vi "Word_auto_text_entry (for page number).vi"(0 "Word._Document in":refnum<k7>, 7 "position (footers)":u16(ring) items=["footers", "headers"], 11 "error in (no error)":errorcluster, 12 "alignment (right)":u16(ring)=2 items=["left", "center", "right"]) -> (4 "Word._Document out":refnum<k7>, 15 "error out":errorcluster)   [LabVIEW 2020, in "NI_ReportGenerationToolkit.lvlib"]
uses:
  <vilib>/addons/_office/NI_ReportGenerationToolkit.lvlib
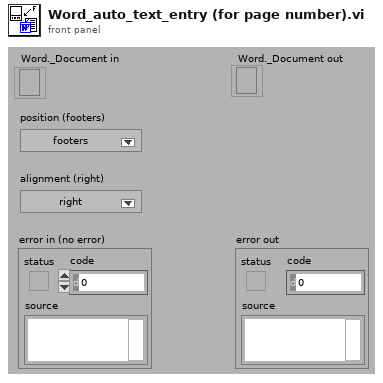
[diagram p1: front panel]
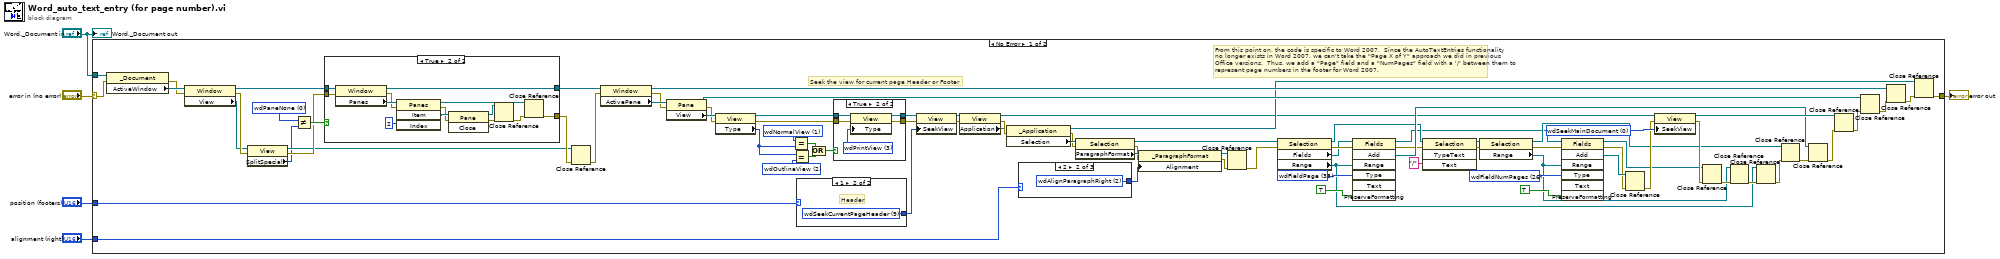
[diagram p0: block diagram]
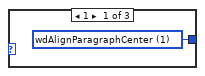
[diagram p2: hidden frame]
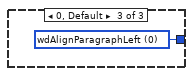
[diagram p3: hidden frame]
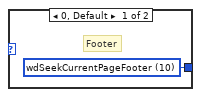
[diagram p4: hidden frame]
diagram:
  n1 = case shown="No Error" "error in (no error)" {
    selector: "error in (no error)" -> [w42 w115]
    tunnel: "Word._Document in" -> [w87 _]
    tunnel: "position (footers)" -> [w58 _]
    tunnel: [w43 w115] -> w4
    tunnel: "alignment (right)" -> [w6 _]
    frame No Error {
      w24 = 26 items=["wdFieldEmpty"=-1, "wdFieldRef"=3, "wdFieldIndexEntry"=4, "wdFieldFootnoteRef"=5, "wdFieldSet"=6, "wdFieldIf"=7, "wdFieldIndex"=8, "wdFieldTOCEntry"=9, "wdFieldStyleRef"=10, "wdFieldRefDoc"=11, "wdFieldSequence"=12, "wdFieldTOC"=13, "wdFieldInfo"=14, "wdFieldTitle"=15, "wdFieldSubject"=16, "wdFieldAuthor"=17, "wdFieldKeyWord"=18, "wdFieldComments"=19, "wdFieldLastSavedBy"=20, "wdFieldCreateDate"=21, "wdFieldSaveDate"=22, "wdFieldPrintDate"=23, "wdFieldRevisionNum"=24, "wdFieldEditTime"=25, "wdFieldNumPages"=26, "wdFieldNumWords"=27, "wdFieldNumChars"=28, "wdFieldFileName"=29, "wdFieldTemplate"=30, "wdFieldDate"=31, "wdFieldTime"=32, "wdFieldPage"=33, "wdFieldExpression"=34, "wdFieldQuote"=35, "wdFieldInclude"=36, "wdFieldPageRef"=37, "wdFieldAsk"=38, "wdFieldFillIn"=39, "wdFieldData"=40, "wdFieldNext"=41, "wdFieldNextIf"=42, "wdFieldSkipIf"=43, "wdFieldMergeRec"=44, "wdFieldDDE"=45, "wdFieldDDEAuto"=46, "wdFieldGlossary"=47, "wdFieldPrint"=48, "wdFieldFormula"=49, "wdFieldGoToButton"=50, "wdFieldMacroButton"=51, "wdFieldAutoNumOutline"=52, "wdFieldAutoNumLegal"=53, "wdFieldAutoNum"=54, "wdFieldImport"=55, "wdFieldLink"=56, "wdFieldSymbol"=57, "wdFieldEmbed"=58, "wdFieldMergeField"=59, "wdFieldUserName"=60, "wdFieldUserInitials"=61, "wdFieldUserAddress"=62, "wdFieldBarCode"=63, "wdFieldDocVariable"=64, "wdFieldSection"=65, "wdFieldSectionPages"=66, "wdFieldIncludePicture"=67, "wdFieldIncludeText"=68, "wdFieldFileSize"=69, "wdFieldFormTextInput"=70, "wdFieldFormCheckBox"=71, "wdFieldNoteRef"=72, "wdFieldTOA"=73, "wdFieldTOAEntry"=74, "wdFieldMergeSeq"=75, "wdFieldPrivate"=77, "wdFieldDatabase"=78, "wdFieldAutoText"=79, "wdFieldCompare"=80, "wdFieldAddin"=81, "wdFieldSubscriber"=82, "wdFieldFormDropDown"=83, "wdFieldAdvance"=84, "wdFieldDocProperty"=85, "wdFieldOCX"=87, "wdFieldHyperlink"=88, "wdFieldAutoTextList"=89, "wdFieldListNum"=90, "wdFieldHTMLActiveX"=91, "wdFieldBidiOutline"=92, "wdFieldAddressBlock"=93, "wdFieldGreetingLine"=94, "wdFieldShape"=95, "wdFieldCitation"=96, "wdFieldBibliography"=97] ("Type")
      w18 = 33 items=["wdFieldEmpty"=-1, "wdFieldRef"=3, "wdFieldIndexEntry"=4, "wdFieldFootnoteRef"=5, "wdFieldSet"=6, "wdFieldIf"=7, "wdFieldIndex"=8, "wdFieldTOCEntry"=9, "wdFieldStyleRef"=10, "wdFieldRefDoc"=11, "wdFieldSequence"=12, "wdFieldTOC"=13, "wdFieldInfo"=14, "wdFieldTitle"=15, "wdFieldSubject"=16, "wdFieldAuthor"=17, "wdFieldKeyWord"=18, "wdFieldComments"=19, "wdFieldLastSavedBy"=20, "wdFieldCreateDate"=21, "wdFieldSaveDate"=22, "wdFieldPrintDate"=23, "wdFieldRevisionNum"=24, "wdFieldEditTime"=25, "wdFieldNumPages"=26, "wdFieldNumWords"=27, "wdFieldNumChars"=28, "wdFieldFileName"=29, "wdFieldTemplate"=30, "wdFieldDate"=31, "wdFieldTime"=32, "wdFieldPage"=33, "wdFieldExpression"=34, "wdFieldQuote"=35, "wdFieldInclude"=36, "wdFieldPageRef"=37, "wdFieldAsk"=38, "wdFieldFillIn"=39, "wdFieldData"=40, "wdFieldNext"=41, "wdFieldNextIf"=42, "wdFieldSkipIf"=43, "wdFieldMergeRec"=44, "wdFieldDDE"=45, "wdFieldDDEAuto"=46, "wdFieldGlossary"=47, "wdFieldPrint"=48, "wdFieldFormula"=49, "wdFieldGoToButton"=50, "wdFieldMacroButton"=51, "wdFieldAutoNumOutline"=52, "wdFieldAutoNumLegal"=53, "wdFieldAutoNum"=54, "wdFieldImport"=55, "wdFieldLink"=56, "wdFieldSymbol"=57, "wdFieldEmbed"=58, "wdFieldMergeField"=59, "wdFieldUserName"=60, "wdFieldUserInitials"=61, "wdFieldUserAddress"=62, "wdFieldBarCode"=63, "wdFieldDocVariable"=64, "wdFieldSection"=65, "wdFieldSectionPages"=66, "wdFieldIncludePicture"=67, "wdFieldIncludeText"=68, "wdFieldFileSize"=69, "wdFieldFormTextInput"=70, "wdFieldFormCheckBox"=71, "wdFieldNoteRef"=72, "wdFieldTOA"=73, "wdFieldTOAEntry"=74, "wdFieldMergeSeq"=75, "wdFieldPrivate"=77, "wdFieldDatabase"=78, "wdFieldAutoText"=79, "wdFieldCompare"=80, "wdFieldAddin"=81, "wdFieldSubscriber"=82, "wdFieldFormDropDown"=83, "wdFieldAdvance"=84, "wdFieldDocProperty"=85, "wdFieldOCX"=87, "wdFieldHyperlink"=88, "wdFieldAutoTextList"=89, "wdFieldListNum"=90, "wdFieldHTMLActiveX"=91, "wdFieldBidiOutline"=92, "wdFieldAddressBlock"=93, "wdFieldGreetingLine"=94, "wdFieldShape"=95, "wdFieldCitation"=96, "wdFieldBibliography"=97] ("Type")
      w55 = 0 items=["wdSeekMainDocument", "wdSeekPrimaryHeader", "wdSeekFirstPageHeader", "wdSeekEvenPagesHeader", "wdSeekPrimaryFooter", "wdSeekFirstPageFooter", "wdSeekEvenPagesFooter", "wdSeekFootnotes", "wdSeekEndnotes", "wdSeekCurrentPageHeader", "wdSeekCurrentPageFooter"] ("SeekView")
      w69 = 2 items=["wdNormalView"=1, "wdOutlineView"=2, "wdPrintView"=3, "wdPrintPreview"=4, "wdMasterView"=5, "wdWebView"=6] ("Type")
      w71 = 1 items=["wdNormalView"=1, "wdOutlineView"=2, "wdPrintView"=3, "wdPrintPreview"=4, "wdMasterView"=5, "wdWebView"=6] ("Type")
      w56 = 0 items=["wdPaneNone", "wdPanePrimaryHeader", "wdPaneFirstPageHeader", "wdPaneEvenPagesHeader", "wdPanePrimaryFooter", "wdPaneFirstPageFooter", "wdPaneEvenPagesFooter", "wdPaneFootnotes", "wdPaneEndnotes", "wdPaneFootnoteContinuationNotice", "wdPaneFootnoteContinuationSeparator", "wdPaneFootnoteSeparator", "wdPaneEndnoteContinuationNotice", "wdPaneEndnoteContinuationSeparator", "wdPaneEndnoteSeparator", "wdPaneComments", "wdPaneCurrentPageHeader", "wdPaneCurrentPageFooter", "wdPaneRevisions"] ("SplitSpecial")
      # "From this point on, the code is specific to Word 2007.  Since the AutoTextEntries functionality no longer exists in Word 2007, we can't take the \"Page X of Y\" approach we did in previous Office versions.  Thus, we add a \"Page\" field and a \"NumPages\" field with a '/' between them to represent page numbers in the footer for Word 2007."
      # "Seek the view for current page Header or Footer"
      n2 = property class="_Document"(reference=w87, error in=w42) -> (error out=w85:errorcluster, "ActiveWindow"=w86:refnum<k7>)  [unwired: 1 out]
      n3 = property class="Window"(reference=w86, error in=w85) -> (reference out=w81:refnum<k7>, error out=w84:errorcluster, "View"=w82:refnum<k7>)
      n4 = property class="View"(reference=w82, error in=w84) -> (reference out=w78:refnum<k7>, error out=w80:errorcluster, "SplitSpecial"=w57:i32)
      n5 = Not Equal?(x=w56, y=w57) -> (x != y?=w83:bool)
      n6 = case shown="True" w83 {
        tunnel: [w100 w104] -> w79
        tunnel: w81 -> [w101 w108]
        tunnel: w80 -> [w100 w105]
        tunnel: [w101 w103] -> w77
        frame False {
        }
        frame True {
          n7 = property class="Window"(reference=w108, error in=w105) -> (reference out=w103:refnum<k7>, error out=w106:errorcluster, "Panes"=w107:refnum<k7>)
          n8 = invoke class="Panes" method="Item"(reference=w107, error in=w106, "Index"=2) -> (reference out=w102:refnum<k7>, error out=w112:errorcluster, "Item"=w113:refnum<k7>)  [unwired: 1 in, 1 out]
          n9 = invoke class="Pane" method="Close"(reference=w113, error in=w112) -> (reference out=w110:refnum<k7>, error out=w111:errorcluster)  [unwired: 1 in, 1 out]
          n10 = Close Reference(reference=w110, error in (no error)=w111) -> (error out=w109:errorcluster)
          n11 = Close Reference(reference=w102, error in (no error)=w109) -> (error out=w104:errorcluster)
        }
      }
      n12 = Close Reference(reference=w78, error in (no error)=w79) -> (error out=w76:errorcluster)
      n13 = property class="Window"(reference=w77, error in=w76) -> (reference out=w46:refnum<k7>, error out=w74:errorcluster, "ActivePane"=w75:refnum<k7>)
      n14 = property class="Pane"(reference=w75, error in=w74) -> (reference out=w48:refnum<k7>, error out=w72:errorcluster, "View"=w73:refnum<k7>)
      n15 = property class="View"(reference=w73, error in=w72) -> (reference out=w65:refnum<k7>, error out=w64:errorcluster, "Type"=w70:i32)
      n16 = Equal?(x=w71, y=w70) -> (x = y?=w67:bool)
      n17 = Equal?(x=w70, y=w69) -> (x = y?=w68:bool)
      n18 = case shown="1" w58 {
        tunnel: [w91 w92] -> w40
        frame 0, Default {
          w91 = 10 items=["wdSeekMainDocument", "wdSeekPrimaryHeader", "wdSeekFirstPageHeader", "wdSeekEvenPagesHeader", "wdSeekPrimaryFooter", "wdSeekFirstPageFooter", "wdSeekEvenPagesFooter", "wdSeekFootnotes", "wdSeekEndnotes", "wdSeekCurrentPageHeader", "wdSeekCurrentPageFooter"] ("SeekView")
          # "Footer"
        }
        frame 1 {
          w92 = 9 items=["wdSeekMainDocument", "wdSeekPrimaryHeader", "wdSeekFirstPageHeader", "wdSeekEvenPagesHeader", "wdSeekPrimaryFooter", "wdSeekFirstPageFooter", "wdSeekEvenPagesFooter", "wdSeekFootnotes", "wdSeekEndnotes", "wdSeekCurrentPageHeader", "wdSeekCurrentPageFooter"] ("SeekView")
          # "Header"
        }
      }
      n19 = Or(x=w67, y=w68) -> (x .or. y?=w66:bool)
      n20 = case shown="True" w66 {
        tunnel: w65 -> [w94 w99]
        tunnel: w64 -> [w93 w98]
        tunnel: [w94 w96] -> w63
        tunnel: [w93 w95] -> w62
        frame False {
        }
        frame True {
          w97 = 3 items=["wdNormalView"=1, "wdOutlineView"=2, "wdPrintView"=3, "wdPrintPreview"=4, "wdMasterView"=5, "wdWebView"=6] ("Type")
          n21 = property class="View"(reference=w99, error in=w98, "Type"=w97) -> (reference out=w96:refnum<k7>, error out=w95:errorcluster)
        }
      }
      n22 = property class="View"(reference=w63, error in=w62, "SeekView"=w40) -> (reference out=w41:refnum<k7>, error out=w61:errorcluster)
      n23 = property class="View"(reference=w41, error in=w61) -> (reference out=w29:refnum<k7>, error out=w60:errorcluster, "Application"=w59:refnum<k7>)
      n24 = property class="_Application"(reference=w59, error in=w60) -> (reference out=w44:refnum<k7>, error out=w14:errorcluster, "Selection"=w15:refnum<k7>)
      n25 = case shown="2" w6 {
        tunnel: [w88 w89 w90] -> w7
        frame 1 {
          w88 = 1 items=["wdAlignParagraphLeft"=0, "wdAlignParagraphCenter"=1, "wdAlignParagraphRight"=2, "wdAlignParagraphJustify"=3, "wdAlignParagraphDistribute"=4, "wdAlignParagraphJustifyMed"=5, "wdAlignParagraphJustifyHi"=7, "wdAlignParagraphJustifyLow"=8, "wdAlignParagraphThaiJustify"=9] ("Alignment")
        }
        frame 2 {
          w89 = 2 items=["wdAlignParagraphLeft"=0, "wdAlignParagraphCenter"=1, "wdAlignParagraphRight"=2, "wdAlignParagraphJustify"=3, "wdAlignParagraphDistribute"=4, "wdAlignParagraphJustifyMed"=5, "wdAlignParagraphJustifyHi"=7, "wdAlignParagraphJustifyLow"=8, "wdAlignParagraphThaiJustify"=9] ("Alignment")
        }
        frame 0, Default {
          w90 = 0 items=["wdAlignParagraphLeft"=0, "wdAlignParagraphCenter"=1, "wdAlignParagraphRight"=2, "wdAlignParagraphJustify"=3, "wdAlignParagraphDistribute"=4, "wdAlignParagraphJustifyMed"=5, "wdAlignParagraphJustifyHi"=7, "wdAlignParagraphJustifyLow"=8, "wdAlignParagraphThaiJustify"=9] ("Alignment")
        }
      }
      n26 = property class="Selection"(reference=w15, error in=w14) -> (reference out=w8:refnum<k7>, error out=w12:errorcluster, "ParagraphFormat"=w13:refnum<k7>)
      n27 = property class="_ParagraphFormat"(reference=w13, error in=w12, "Alignment"=w7) -> (reference out=w10:refnum<k7>, error out=w11:errorcluster)
      n28 = Close Reference(reference=w10, error in (no error)=w11) -> (error out=w9:errorcluster)
      n29 = property class="Selection"(reference=w8, error in=w9) -> (reference out=w25:refnum<k7>, error out=w39:errorcluster, "Fields"=w37:refnum<k7>, "Range"=w16:refnum<k7>)
      n30 = invoke class="Fields" method="Add"(reference=w37, error in=w39, "Range"=w16, "Type"=w18, "PreserveFormatting"=TRUE) -> (reference out=w22:refnum<k7>, error out=w21:errorcluster, "Add"=w33:refnum<k7>)  [unwired: 2 in, 4 out]
      n31 = invoke class="Selection" method="TypeText"(reference=w25, error in=w21, "Text"="/") -> (reference out=w31:refnum<k7>, error out=w32:errorcluster)  [unwired: 1 in, 2 out]
      n32 = property class="Selection"(reference=w31, error in=w32) -> (reference out=w23:refnum<k7>, error out=w30:errorcluster, "Range"=w17:refnum<k7>)
      n33 = invoke class="Fields" method="Add"(reference=w22, error in=w30, "Range"=w17, "Type"=w24, "PreserveFormatting"=TRUE) -> (reference out=w19:refnum<k7>, error out=w20:errorcluster, "Add"=w34:refnum<k7>)  [unwired: 2 in, 4 out]
      n34 = Close Reference(reference=w34, error in (no error)=w20) -> (error out=w54:errorcluster)
      n35 = property class="View"(reference=w29, error in=w54, "SeekView"=w55) -> (reference out=w52:refnum<k7>, error out=w53:errorcluster)
      n36 = Close Reference(reference=w19, error in (no error)=w53) -> (error out=w28:errorcluster)
      n37 = Close Reference(reference=w17, error in (no error)=w28) -> (error out=w27:errorcluster)
      n38 = Close Reference(reference=w16, error in (no error)=w27) -> (error out=w26:errorcluster)
      n39 = Close Reference(reference=w23, error in (no error)=w26) -> (error out=w51:errorcluster)
      n40 = Close Reference(reference=w33, error in (no error)=w51) -> (error out=w50:errorcluster)
      n41 = Close Reference(reference=w52, error in (no error)=w50) -> (error out=w49:errorcluster)
      n42 = Close Reference(reference=w48, error in (no error)=w49) -> (error out=w47:errorcluster)
      n43 = Close Reference(reference=w46, error in (no error)=w47) -> (error out=w45:errorcluster)
      n44 = Close Reference(reference=w44, error in (no error)=w45) -> (error out=w43:errorcluster)
    }
    frame Error {
    }
  }
  "error out" <- w4
  "Word._Document out" <- "Word._Document in"
